vi "SetV.vi"(8 "error in (no error)":errorcluster, 10 "test":dbl, 11 "axopatch-200B in":refnum<class "axopatch-200B.lvclass">) -> (0 "error out":errorcluster, 3 "axopatch-200B out":refnum<class "axopatch-200B.lvclass">)   [LabVIEW 2014, in "axopatch-200B.lvclass"]
uses:
  axopatch-200B.lvclass
  axopatch-200B.lvclass/axopatch-200B.ctl
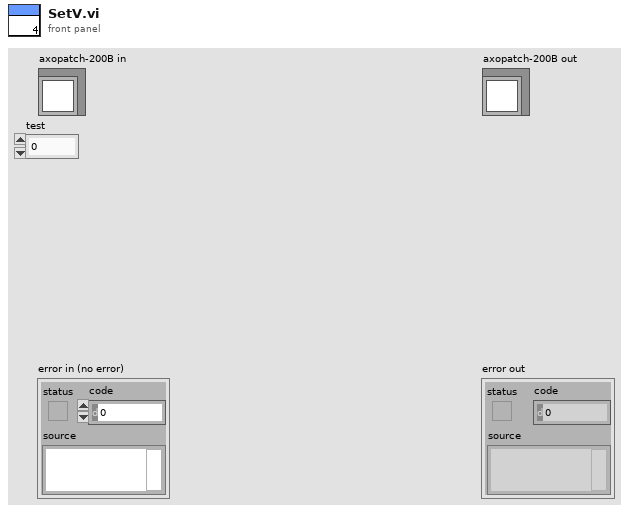
[diagram p1: front panel]
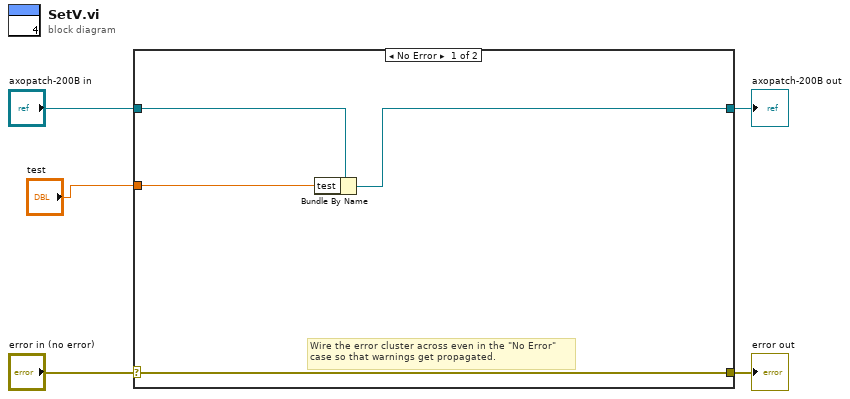
[diagram p0: block diagram]
diagram:
  n1 = case shown="No Error" "error in (no error)" {
    selector: "error in (no error)" -> [w9 w11]
    tunnel: [w9 w11] -> w4
    tunnel: [w7 w10] -> w2
    tunnel: "axopatch-200B in" -> [w8 w10]
    tunnel: "test" -> [w6 _]
    frame No Error {
      # "Wire the error cluster across even in the \"No Error\"\ncase so that warnings get propagated."
      n2 = Bundle By Name(cluster=w8, "test"=w6) -> (w7:refnum<class "axopatch-200B.lvclass">)
    }
    frame Error {
    }
  }
  "error out" <- w4
  "axopatch-200B out" <- w2
